vi "Update Value.vi"(6 "Time":dbl, 8 "error in (no error)":errorcluster, 11 "DoubleControl in":refnum<class "SliderControl.lvclass">) -> (0 "error out":errorcluster, 1 "Update":bool, 2 "Value":variant, 3 "DoubleControl out":refnum<class "SliderControl.lvclass">)   [LabVIEW 2020, in "VolatusGUIElements.lvlib" / "SliderControl.lvclass"]
uses:
  SliderControl.lvclass
  SliderControl.lvclass/SliderControl.ctl
  lv-vecto/Vecto/Channel DBL/Channel DBL.lvclass/Channel DBL.ctl
  lv-vecto/Vecto/Group DBL/Value by Index.vi
  lv-vecto/Vecto/Channel DBL/Channel DBL.lvclass
  VolatusGUIElements.lvlib
  VolatusGUI/Element Inhibit/Element Inhibit.lvclass
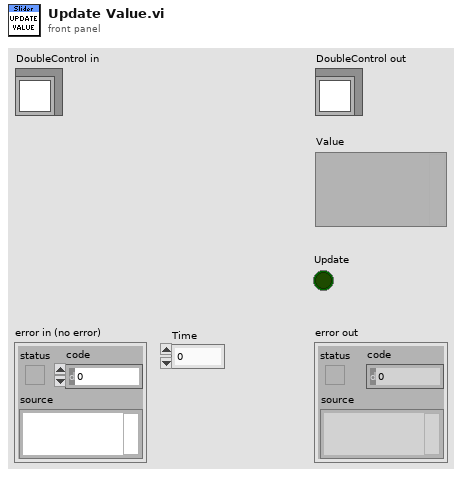
[diagram p1: front panel]
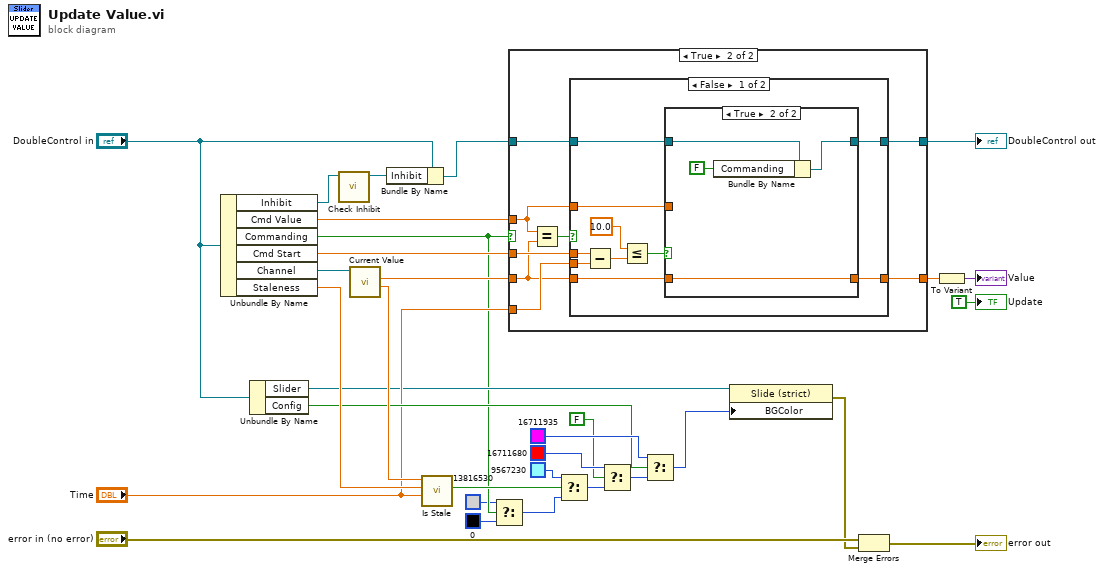
[diagram p0: block diagram]
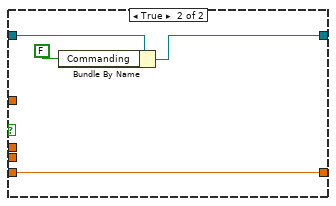
[diagram p4: hidden frame]
diagram:
  n1 = Unbundle By Name("DoubleControl in") -> ("Inhibit"=w3:refnum<class "Element Inhibit.lvclass">, "Cmd Value"=w19:dbl, "Commanding"=w5:bool, "Cmd Start"=w27:dbl, "Channel"=w31:refnum<class "Channel DBL.lvclass">, "Staleness"=w29:dbl)
  n2 = Unbundle By Name("DoubleControl in") -> ("Slider"=w11:refnum<vi>, "Config"=w20:bool)
  n3 = call "Check Inhibit.vi"("Element Inhibit in"=w3) -> ("Element Inhibit out"=w1:refnum<class "Element Inhibit.lvclass">)  [unwired: 9 in, 1 out]
  n4 = call "Current Value.vi"("Channel in"=w31) -> ("Timestamp"=w30:dbl, "Scaled"=w28:dbl)  [unwired: 6 in, 3 out]
  n5 = Bundle By Name(cluster="DoubleControl in", "Inhibit"=w1) -> (w2:refnum<class "SliderControl.lvclass">)
  n6 = call "Is Stale.vi"("Time"="Time", "Staleness"=w29, "Timestamp"=w30) -> ("Stale"=w26:bool)  [unwired: 8 in]
  n7 = Select(t=u32 13816530, s=w5, f=u32 0) -> (s? t:f=w6:u32)
  n8 = case shown="True" w5 {
    tunnel: w28 -> [w34 w39]
    tunnel: w27 -> [_ w42]
    tunnel: "Time" -> [_ w41]
    tunnel: w19 -> [_ w35]
    tunnel: w2 -> [w33 w38]
    tunnel: [w33 w37] -> w18
    tunnel: [w34 w36] -> w15
    frame False {
    }
    frame True {
      n9 = Equal?(x=w35, y=w39) -> (x = y?=w40:bool)
      n10 = case shown="False" w40 {
        tunnel: w42 -> [w52 _]
        tunnel: w41 -> [w51 _]
        tunnel: w39 -> [w45 w59]
        tunnel: w38 -> [w47 w62]
        tunnel: [w46 w60] -> w37
        tunnel: [w43 w59] -> w36
        tunnel: w35 -> [w44 _]
        frame False {
          n11 = Subtract(x=w52, y=w51) -> (x-y=w50:dbl)
          n12 = Less Or Equal?(x=10.0, y=w50) -> (x <= y?=w48:bool)
          n13 = case shown="True" w48 {
            tunnel: w47 -> [w53 w58]
            tunnel: [w53 w56] -> w46
            tunnel: w45 -> [_ w55]
            tunnel: w44 -> [w54 _]
            tunnel: [w54 w55] -> w43
            frame False {
            }
            frame True {
              n14 = Bundle By Name(cluster=w58, "Commanding"=FALSE) -> (w56:refnum<class "SliderControl.lvclass">)
            }
          }
        }
        frame True {
          n15 = Bundle By Name(cluster=w62, "Commanding"=FALSE) -> (w60:refnum<class "SliderControl.lvclass">)
        }
      }
    }
  }
  "DoubleControl out" <- w18
  n16 = Select(t=u32 9567230, s=w26, f=w6) -> (s? t:f=w24:u32)
  n17 = Select(t=u32 16711680, s=FALSE, f=w24) -> (s? t:f=w22:u32)
  n18 = Select(t=u32 16711935, s=w20, f=w22) -> (s? t:f=w10:u32)
  n19 = property class="Slide (strict)"(reference=w11, "BGColor"=w10) -> (error out=w8:errorcluster)  [unwired: 1 in, 1 out]
  n20 = Merge Errors("error in (no error)", w8) -> (→"error out":errorcluster)
  n21 = To Variant(anything=w15) -> (Variant=→"Value":variant)
  "Update" <- TRUE ("Update")
